vi "filtra mei.vi"(0 "Array":string[](array[string])) -> (12 "indici grafici m,3,6 mei":T1[](array[typedef]), 14 "Array Array 1ph out":string[](array[string]), 15 "Array 3ph3ch out":string[](array[string]), 16 "Array 3ph6ch out":string[](array[string]), 17 "Incerterzza m":string[](array[string]), 18 "Incertezza 3":string[](array[string]), 19 "Incertezza 6":string[](array[string]))   [LabVIEW 2019]
uses:
  TypeDef/Indici.ctl
  <vilib>/Utility/file.llb/Read From Spreadsheet File (string).vi
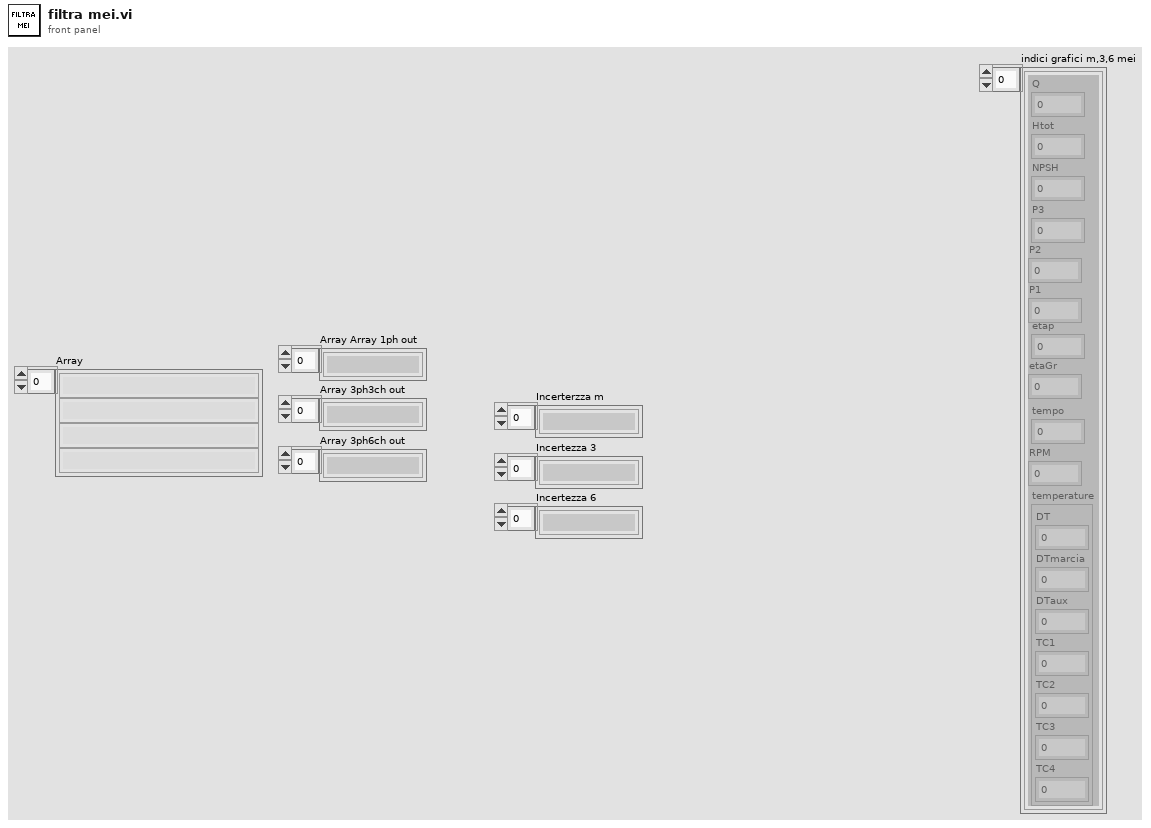
[diagram p1: front panel]
types:
  T1 = typedef "Indici.ctl" = cluster{"Q":i32, "Htot":i32, "NPSH":i32, "P3":i32, "etap":i32, "temperature":cluster{"DT":i32, "DTmarcia":i32, "DTaux":i32, "TC1":i32, "TC2":i32, "TC3":i32, "TC4":i32}, "tempo":i32, "P2":i32, "P1":i32, "etaGr":i32, "RPM":i32}
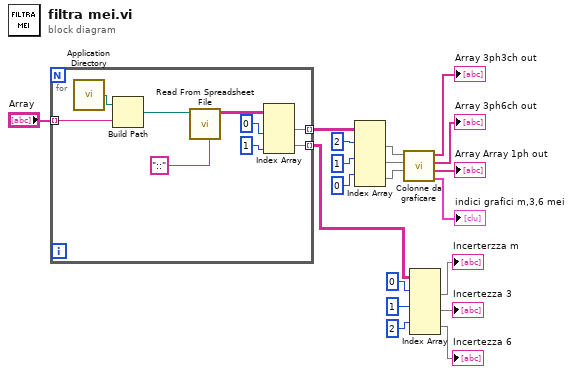
[diagram p0: block diagram]
diagram:
  n1 = for {
    tunnel: "Array" -> [w25] mode=indexing
    tunnel: [w21] -> w19 mode=indexing
    tunnel: [w20] -> w5 mode=indexing
    n2 = call <vilib>:"Application Directory.vi"() -> ("Application Directory"=w28:path)
    n3 = Build Path(base path=w28, name or relative path=w25) -> (appended path=w27:path)
    n4 = call-poly <vilib>:"Read From Spreadsheet File.vi"("delimiter (\\t)"="::" ("delimiter (\\t)"), "file path (dialog if empty)"=w27) -> ("all rows"=w22:string[][])  [unwired: 5 in, 4 out]
    n5 = Index Array(array=w22, index (col) #1=0 ("disabled index (col)"), index (col) #2=1 ("index (col)")) -> (element #1=w21:string[], element #2=w20:string[])  [unwired: 2 in]
  }
  n6 = Index Array(array=w19, index (row) #1=2 ("index (row)"), index (row) #2=1 ("index (row)"), index (row) #3=0 ("index (row)")) -> (element #1=w14:string[], element #2=w13:string[], element #3=w12:string[])  [unwired: 3 in]
  n7 = call "Colonne da graficare.vi"("Array 1ph"=w12, "Array 3ph6ch"=w13, "Array 3ph3ch"=w14) -> ("indici grafici m,3,6"=→"indici grafici m,3,6 mei":T1[], "Array Array 1ph out"=→"Array Array 1ph out":string[], "Array 3ph6ch out"=→"Array 3ph6ch out":string[], "Array 3ph3ch out"=→"Array 3ph3ch out":string[])  [unwired: 4 in]
  n8 = Index Array(array=w5, index (row) #1=0 ("index (row)"), index (row) #2=1 ("index (row)"), index (row) #3=2 ("index (row)")) -> (element #1=→"Incerterzza m":string[], element #2=→"Incertezza 3":string[], element #3=→"Incertezza 6":string[])  [unwired: 3 in]
